vi "midiOutGetDevCapsA.vi"(8 "error in":errorcluster, 10 "DeviceID":u32, 11 "midi in":refnum<class "midi.lvclass">) -> (0 "error out":errorcluster, 3 "midi out":refnum<class "midi.lvclass">)   [LabVIEW 2020, in "midi.lvclass"]
uses:
  midi.lvclass
  midi.lvclass/midi.ctl
  winmm.dll
panel:
  out "cbmoc":u32
  out "pmoc":T1
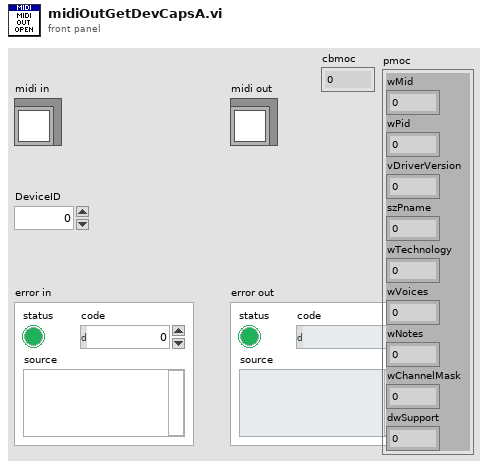
[diagram p1: front panel]
types:
  T1 = cluster{"wMid":u16, "wPid":u16, "vDriverVersion":u16, "szPname":u16, "wTechnology":u16, "wVoices":u16, "wNotes":u16, "wChannelMask":u16, "dwSupport":i32}
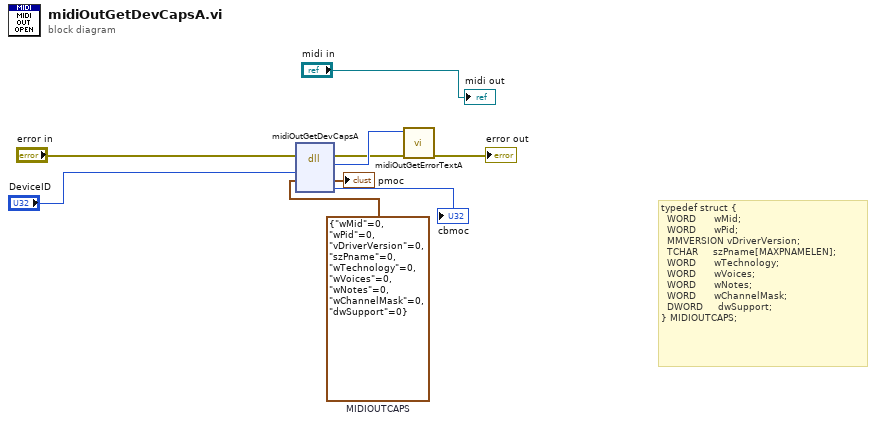
[diagram p0: block diagram]
diagram:
  w3 = T1 {"wMid"=0, "wPid"=0, "vDriverVersion"=0, "szPname"=0, "wTechnology"=0, "wVoices"=0, "wNotes"=0, "wChannelMask"=0, "dwSupport"=0}  # MIDIOUTCAPS
  # "typedef struct {\n  WORD      wMid;\n  WORD      wPid;\n  MMVERSION vDriverVersion;\n  TCHAR     szPname[MAXPNAMELEN];\n  WORD      wTechnology;\n  WORD      wVoices;\n  WORD      wNotes;\n  WORD      wChannelMask;\n  DWORD     dwSupport;\n} MIDIOUTCAPS;"
  n1 = dll-call lib="winmm.dll" fn="midiOutGetDevCapsA"(error in="error in", "uDeviceID"="DeviceID", "pmoc"=w3) -> (error out=w8:errorcluster, "errorcode"=w9:i32, "pmoc"=→"pmoc":T1, "cbmoc"=→"cbmoc":u32)  [unwired: 4 in, 1 out]
  n2 = call "midiOutGetErrorTextA.vi"("error in"=w8, "Error Code"=w9) -> ("error out"=→"error out":errorcluster)  [unwired: 9 in]
  "midi out" <- "midi in"
